vi "RHT Setup (SubVI).vi"(0 "RH Used?":bool[](array[boolean]), 1 "Vaisala T Scale":tag="Vaisala T", 2 "Error In":errorcluster, 3 "TC Used?":bool[](array[boolean]), 4 "RHT (T) Channels":tag[](array[tag]), 5 "Vaisala RH Scale":tag="Vaisala RH", 6 "RH Names":string[](array[string]), 7 "RH Channels":tag[](array[tag]), 11 "RHT (T) Names":string[](array[string])) -> (13 "RH Labels":string[](array[string]), 20 "Refnum out":refnum<k21>, 21 "# RH Probes":i32, 24 "# RH (T) Probes":i32, 25 "RH (T) Labels":string[](array[string]), 27 "error out":errorcluster)   [LabVIEW 2011]
uses:
  <vilib>/Utility/error.llb/DialogType.ctl
  <vilib>/DAQmx/create/channels.llb/DAQmx Create Channel (AI-Voltage-Basic).vi
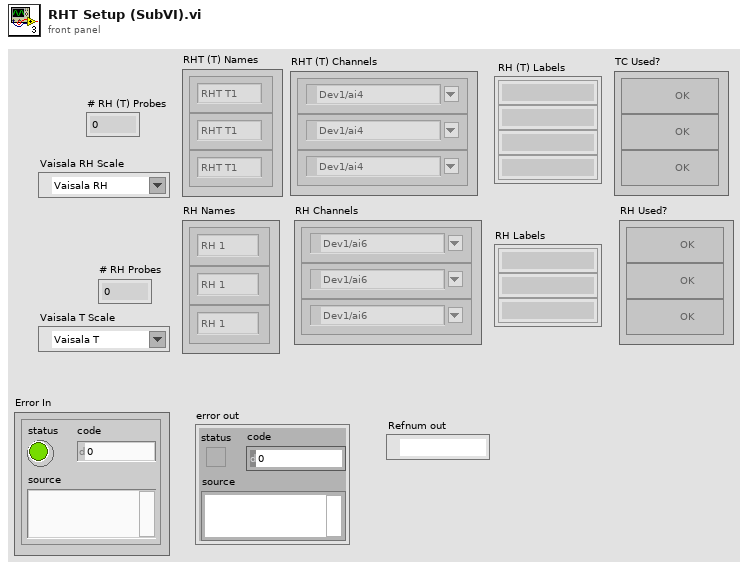
[diagram p1: front panel]
types:
  T1 = typedef "DialogType.ctl" = u16
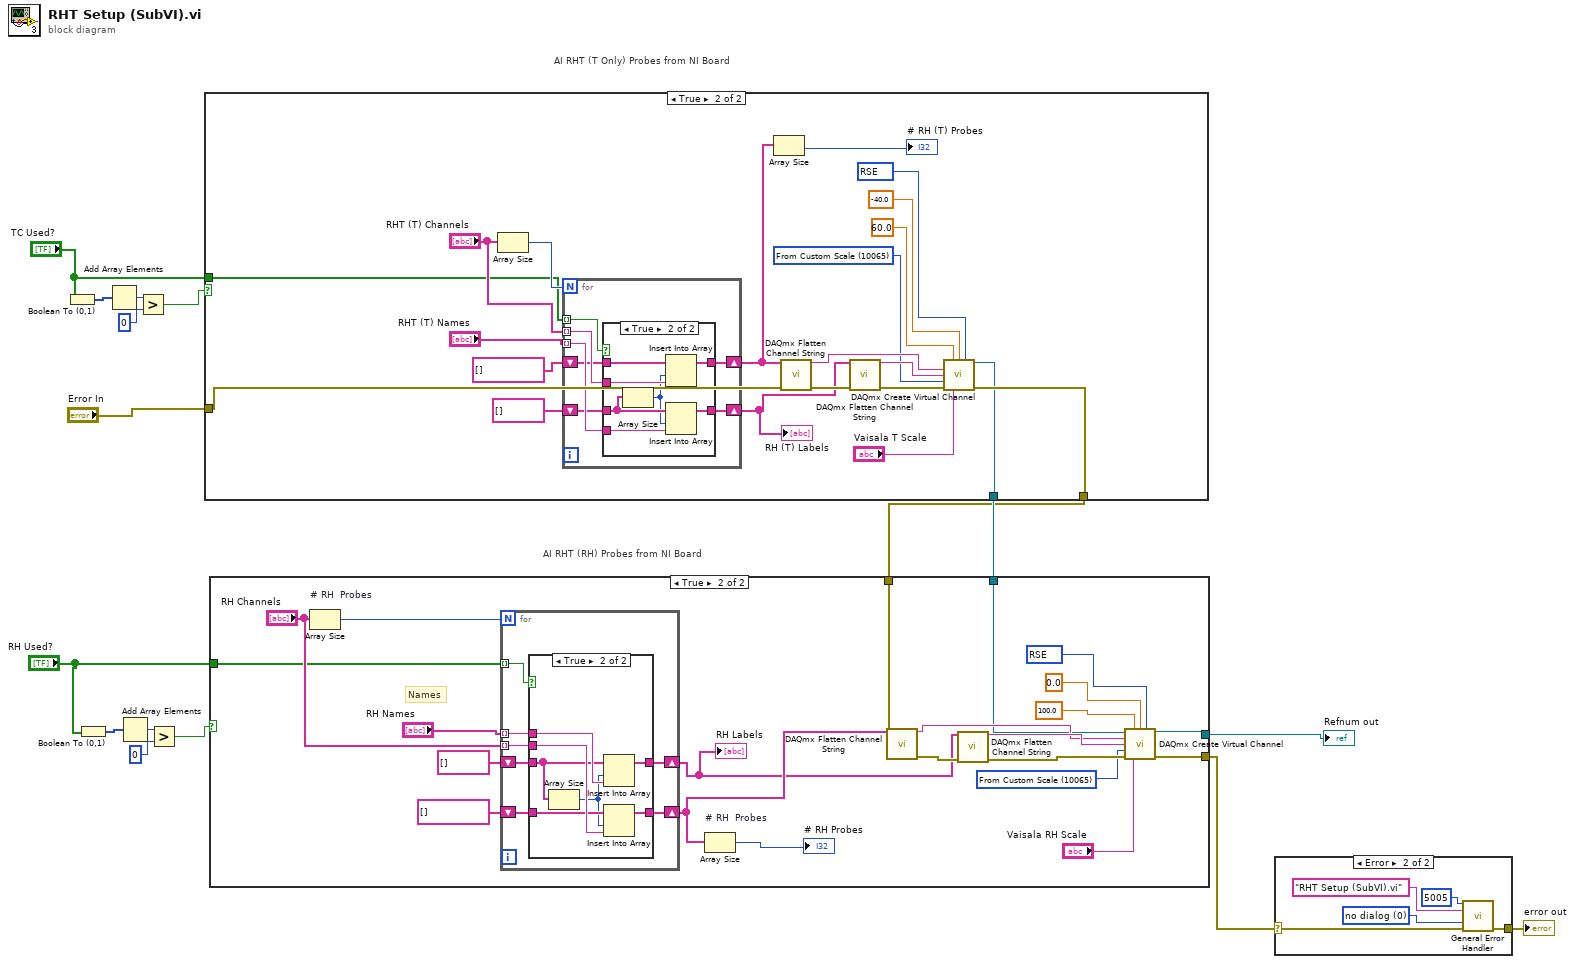
[diagram p0: block diagram]
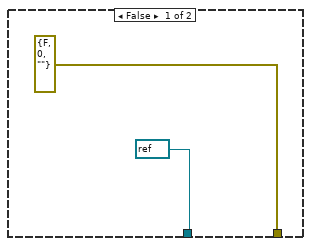
[diagram p3: hidden frame]
diagram:
  # "AI RHT (T Only) Probes from NI Board"
  # "AI RHT (RH) Probes from NI Board"
  n1 = Boolean To (0,1)(Boolean="TC Used?") -> (0, 1=w12:i16[])
  n2 = Boolean To (0,1)(Boolean="RH Used?") -> (0, 1=w16:i16[])
  n3 = Add Array Elements(numeric array=w12) -> (sum=w11:i16)
  n4 = Add Array Elements(numeric array=w16) -> (sum=w15:i16)
  n5 = Greater?(x=w11, y=i16 0) -> (0:w9:bool)
  n6 = Greater?(x=w15, y=i16 0) -> (0:w13:bool)
  n7 = case shown="True" w9 {
    tunnel: [errorcluster {"status"=FALSE, "code"=0, "source"=""} ("error out") w28] -> w7
    tunnel: "TC Used?" -> [_ w25]
    tunnel: [refnum<k21> refnum ("task out") w24] -> w8
    tunnel: "Error In" -> [_ w19]
    frame False {
    }
    frame True {
      w27 = 10083 items=["default"=-1, "RSE"=10083, "NRSE"=10078, "Differential"=10106, "Pseudodifferential"=12529] ("input terminal configuration")
      w32 = 10065 items=["Volts"=10348, "From Custom Scale"=10065] ("units")
      n8 = Array Size(array="RHT (T) Channels") -> (size(s)=w37:i32)
      n9 = for {
        N: w37 -> [_]
        tunnel: w25 -> [w46] mode=indexing
        tunnel: "RHT (T) Channels" -> [w44] mode=indexing
        tunnel: "RHT (T) Names" -> [w45] mode=indexing
        shift-right: [w43] -> w26
        shift-left: tag[] [] -> [w42]
        shift-right: [w41] -> w23
        shift-left: string[] [] -> [w40]
        n10 = case shown="True" w46 {
          tunnel: w45 -> [_ w54]
          tunnel: w44 -> [_ w55]
          tunnel: [w48 w53] -> w43
          tunnel: w42 -> [w48 w52]
          tunnel: [w47 w51] -> w41
          tunnel: w40 -> [w47 w50]
          frame False {
          }
          frame True {
            n11 = Array Size(array=w50) -> (size(s)=w49:i32)
            n12 = Insert Into Array(array=w52, index=w49, new element=w55) -> (w53:tag[])
            n13 = Insert Into Array(array=w50, index=w49, new element=w54) -> (w51:string[])
          }
        }
      }
      "RH (T) Labels" <- w23
      n14 = Array Size(array=w26) -> (size(s)=→"# RH (T) Probes":i32)
      n15 = call <vilib>:"DAQmx Flatten Channel String.vi"("names in"=w26, "error in"=w19) -> ("names out"=w34:string, "error out"=w39:errorcluster)  [unwired: 12 in]
      n16 = call <vilib>:"DAQmx Flatten Channel String.vi"("names in"=w23, "error in"=w39) -> ("names out"=w33:string, "error out"=w29:errorcluster)  [unwired: 12 in]
      n17 = call-poly <vilib>:"DAQmx Create Virtual Channel.vi"("maximum value"=60.0, "minimum value"=-40.0, "input terminal configuration"=w27, "physical channels"=w34, "name to assign"=w33, "units"=w32, "error in"=w29, "custom scale name"="Vaisala T Scale") -> ("task out"=w24:refnum<k21>, "error out"=w28:errorcluster)  [unwired: 6 in]
    }
  }
  n18 = case shown="True" w13 {
    tunnel: "RH Used?" -> [_ w66]
    tunnel: w8 -> [w56 w65]
    tunnel: [w56 w64] -> w6
    tunnel: [w57 w63] -> w2
    tunnel: w7 -> [w57 w62]
    frame False {
    }
    frame True {
      w79 = 10083 items=["default"=-1, "RSE"=10083, "NRSE"=10078, "Differential"=10106, "Pseudodifferential"=12529] ("input terminal configuration")
      w77 = 10065 items=["Volts"=10348, "From Custom Scale"=10065] ("units")
      # "Names"
      n19 = Array Size "# RH  Probes"(array="RH Channels") -> (size(s)=w68:i32)
      n20 = for {
        N: w68 -> [_]
        tunnel: w66 -> [w86] mode=indexing
        tunnel: "RH Channels" -> [w84] mode=indexing
        tunnel: "RH Names" -> [w85] mode=indexing
        shift-right: [w83] -> w67
        shift-left: tag[] [] -> [w82]
        shift-right: [w81] -> w61
        shift-left: string[] [] -> [w80]
        n21 = case shown="True" w86 {
          tunnel: w85 -> [_ w94]
          tunnel: w84 -> [_ w95]
          tunnel: [w88 w93] -> w83
          tunnel: w82 -> [w88 w92]
          tunnel: [w87 w91] -> w81
          tunnel: w80 -> [w87 w90]
          frame False {
          }
          frame True {
            n22 = Array Size(array=w90) -> (size(s)=w89:i32)
            n23 = Insert Into Array(array=w90, index=w89, new element=w94) -> (w91:string[])
            n24 = Insert Into Array(array=w92, index=w89, new element=w95) -> (w93:tag[])
          }
        }
      }
      "RH Labels" <- w61
      n25 = Array Size "# RH  Probes"(array=w67) -> (size(s)=→"# RH Probes":i32)
      n26 = call <vilib>:"DAQmx Flatten Channel String.vi"("names in"=w67, "error in"=w62) -> ("names out"=w75:string, "error out"=w74:errorcluster)  [unwired: 12 in]
      n27 = call <vilib>:"DAQmx Flatten Channel String.vi"("names in"=w61, "error in"=w74) -> ("names out"=w76:string, "error out"=w78:errorcluster)  [unwired: 12 in]
      n28 = call-poly <vilib>:"DAQmx Create Virtual Channel.vi"("task in"=w65, "maximum value"=100.0, "minimum value"=0.0, "input terminal configuration"=w79, "physical channels"=w75, "name to assign"=w76, "units"=w77, "error in"=w78, "custom scale name"="Vaisala RH Scale") -> ("task out"=w64:refnum<k21>, "error out"=w63:errorcluster)  [unwired: 5 in]
    }
  }
  "Refnum out" <- w6
  n29 = case shown="Error" w2 {
    selector: w2 -> [w96 w101]
    tunnel: [w96 w100] -> w1
    frame No Error {
    }
    frame Error {
      w98 = T1 0 items=["no dialog", "OK message", "continue or stop message", "OK message + warnings", "continue/stop + warnings"] ("type of dialog (OK msg:1)")
      n30 = call <vilib>:"General Error Handler.vi"("[error code] (0)"=5005, "[error source] (\" \")"="RHT Setup (SubVI).vi" ("[error source] (\" \")"), "type of dialog (OK msg:1)"=w98, "error in (no error)"=w101) -> ("error out"=w100:errorcluster)  [unwired: 7 in, 4 out]
    }
  }
  "error out" <- w1
